vi "插入数据.vi"(5 "data":variant, 7 "columns":string[](array[string]), 8 "error in (no error)":errorcluster, 10 "database":string, 11 "table":string) -> (0 "error out":errorcluster)   [LabVIEW 2016, in "斯坦道CODMn.lvlib"]
uses:
  <vilib>/addons/database/Connection.llb/DB Tools Open Connec (String).vi
  <vilib>/addons/database/NI_Database_API.lvlib
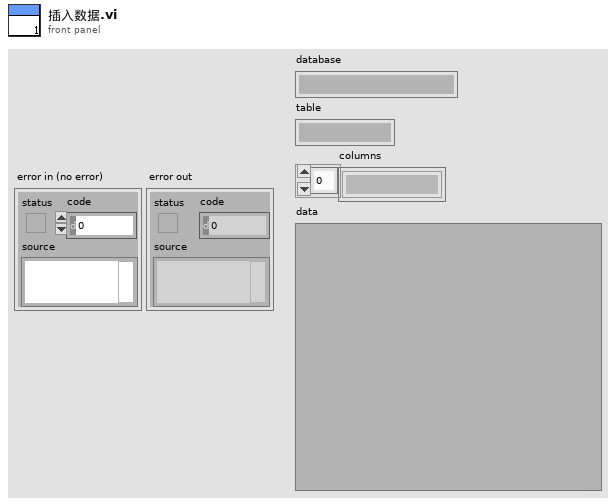
[diagram p1: front panel]
types:
  T1 = typedef "NI_Database_API.lvlib/Conn ObjectReference.ctl" = refnum<k1>
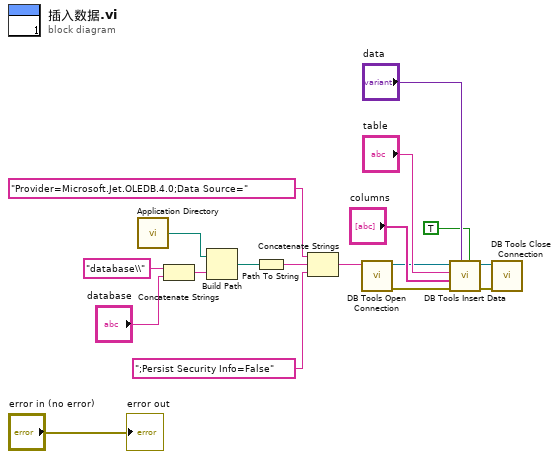
[diagram p0: block diagram]
diagram:
  n1 = call <vilib>:"Application Directory.vi"() -> ("Application Directory"=w1:path)
  n2 = Concatenate Strings("database\\" ("condition"), "database") -> (w7:string)
  n3 = Build Path(base path=w1, name or relative path=w7) -> (appended path=w12:path)
  n4 = Path To String(path=w12) -> (string=w11:string)
  n5 = Concatenate Strings("Provider=Microsoft.Jet.OLEDB.4.0;Data Source=" ("condition"), w11, ";Persist Security Info=False" ("condition")) -> (w9:string)
  n6 = call-poly <vilib>:"DB Tools Open Connection.vi"("connection information"=w9) -> ("error out"=w3:errorcluster, "connection reference"=w4:T1)  [unwired: 7 in]
  n7 = call <vilib>:"DB Tools Insert Data.vi"("create table? (F)"=TRUE, "data"="data", "error in (no error)"=w3, "columns"="columns", "table"="table", "connection reference"=w4) -> ("error out"=w17:errorcluster, "connection reference out"=w18:T1)  [unwired: 4 in]
  n8 = call <vilib>:"DB Tools Close Connection.vi"("error in (no error)"=w17, "connection reference"=w18) -> ()  [unwired: 5 in, 1 out]
  "error out" <- "error in (no error)"
